vi "Set RAM and CPU Channel Properties.vi"(8 "error in (no error)":errorcluster, 10 "Logger Parameters":T1, 11 "Refnum in":refnum<k34>) -> (0 "error out":errorcluster, 3 "Refnum out":refnum<k34>)   [LabVIEW 2019, in "Telemetry Engine.lvlib"]
doc: "This VI sets the Physical Memory and CPU channel information along with their properties."
uses:
  Telemetry Engine.lvlib
  Types/Logger Data.ctl
  Types/Async Logger State Data.ctl
  Types/System Channels.ctl
  Types/Target Info.ctl
  Shared/Constants.vi
  Shared/Telemetry Shared.lvlib
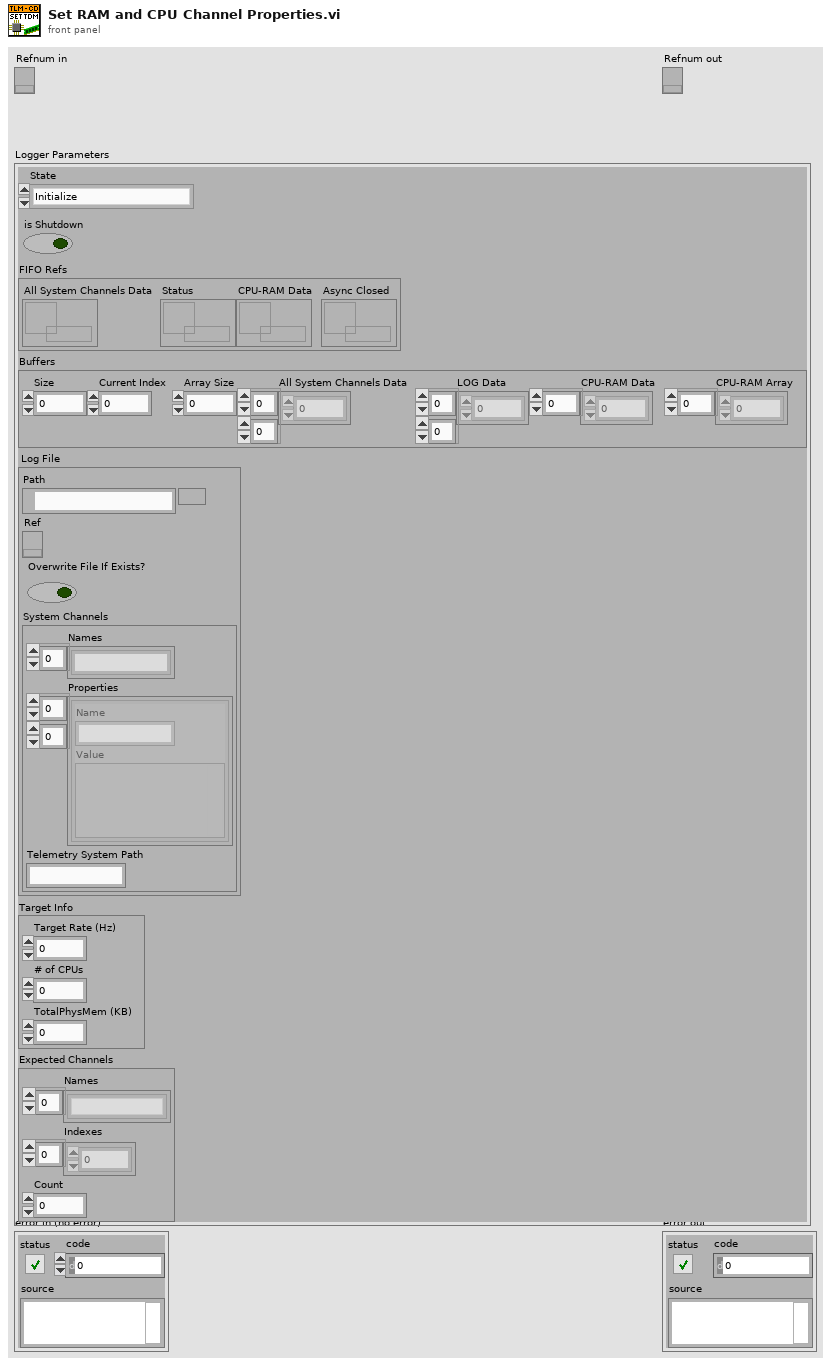
[diagram p1: front panel]
types:
  T1 = typedef "Telemetry Engine.lvlib/Logger Data.ctl" = cluster{"State":T2, "is Shutdown":bool, "FIFO Refs":cluster{"All System Channels Data":refnum<k33>, "Status":refnum<k33>, "CPU-RAM Data":refnum<k33>, "Async Closed":refnum<k33>}, "Buffers":cluster{"Size":i32, "Current Index":i32, "Array Size":i32, "All System Channels Data":dbl[][], "LOG Data":dbl[][], "CPU-RAM Data":dbl[], "CPU-RAM Array":dbl[]}, "Log File":cluster{"Path":path, "Ref":refnum<k34>, "Overwrite File If Exists?":bool, "System Channels":T3}, "Target Info":T4, "Expected Channels":cluster{"Names":string[], "Indexes":i32[], "Count":i32}}
  T2 = typedef "Telemetry Engine.lvlib/Async Logger State Data.ctl" = enum16{"Initialize", "Read System Channels FIFO", "Filter System Channels", "Read CPU-RAM FIFO", "Log Data", "Shutdown"}
  T3 = typedef "Telemetry Engine.lvlib/System Channels.ctl" = cluster{"Names":string[], "Properties":cluster{"Name":string, "Value":variant}[][], "Telemetry System Path":string}
  T4 = typedef "Telemetry Engine.lvlib/Target Info.ctl" = cluster{"Target Rate (Hz)":dbl, "# of CPUs":u32, "TotalPhysMem (KB)":dbl}
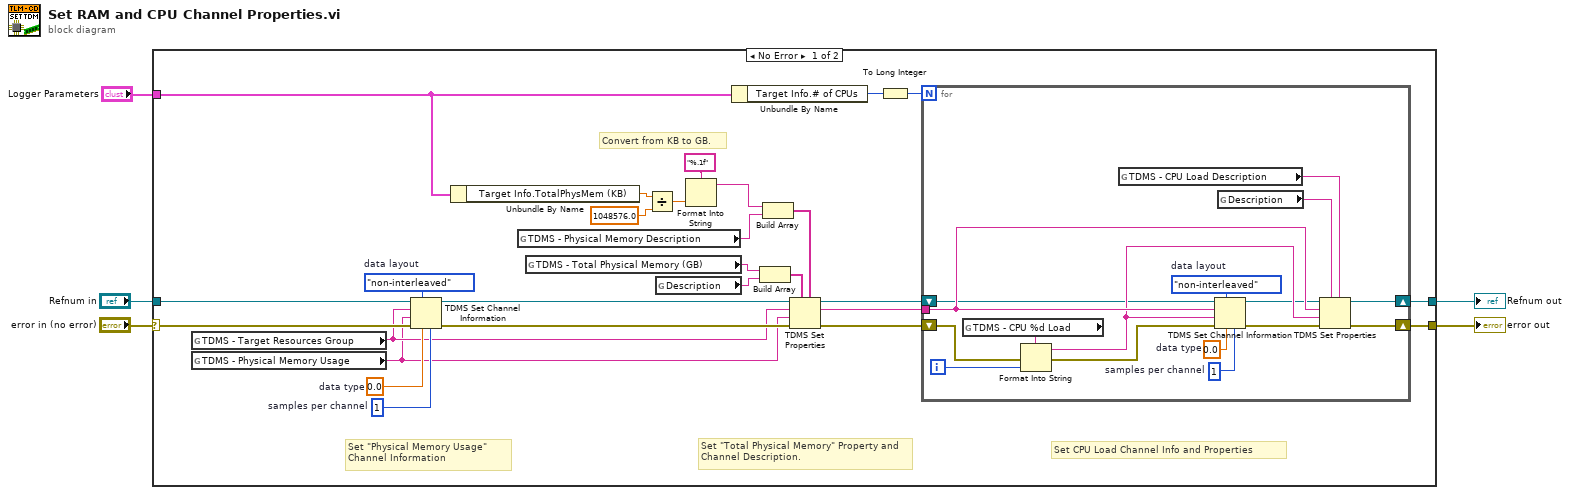
[diagram p0: block diagram]
diagram:
  n1 = case shown="No Error" "error in (no error)" {
    selector: "error in (no error)" -> [w28 w50]
    tunnel: "Logger Parameters" -> [w21 _]
    tunnel: "Refnum in" -> [w26 w49]
    tunnel: [w18 w49] -> w4
    tunnel: [w22 w50] -> w3
    frame No Error {
      w23 = u32 1  # samples per channel
      w24 = 0.0  # data type
      w25 = enum16{"non-interleaved", "interleaved"}."non-interleaved"  # data layout
      # "Set CPU Load Channel Info and Properties"
      # "Set \"Physical Memory Usage\" Channel Information"
      # "Set \"Total Physical Memory\" Property and Channel Description."
      # "Convert from KB to GB."
      n2 = global read "Constants.vi" "TDMS - Target Resources Group"() -> (w7:string)
      n3 = global read "Constants.vi" "TDMS - Physical Memory Usage"() -> (w6:string)
      n4 = TDMS Set Channel Information(4:w23, 6:w24, 7:w25, 8:w28, 9:w6, 10:w7, 11:w26) -> (0:w29:errorcluster, 3:w27:refnum<k34>)
      n5 = Unbundle By Name(w21) -> ("Target Info.TotalPhysMem (KB)"=w31:dbl)
      n6 = global read "Constants.vi" "TDMS - Physical Memory Description"() -> (w11:string)
      n7 = global read "Constants.vi" "TDMS - Total Physical Memory (GB)"() -> (w14:string)
      n8 = Divide(x=w31, y=1048576.0) -> (x/y=w17:dbl)
      n9 = global read "Constants.vi" "Description"() -> (w12:string)
      n10 = Format Into String(format string="%.1f", w17) -> (resulting string=w13:string)  [unwired: 2 in, 1 out]
      n11 = Unbundle By Name(w21) -> ("Target Info.# of CPUs"=w20:u32)
      n12 = Build Array(w14, w12) -> (w15:string[])
      n13 = Build Array(w13, w11) -> (w10:string[])
      n14 = TDMS Set Properties(5:w10, 7:w15, 8:w29, 9:w6, 10:w7, 11:w27) -> (0:w32:errorcluster, 2:w9:string, 3:w8:refnum<k34>)  [unwired: 1 out]
      n15 = To Long Integer(number=w20) -> (32bit integer=w19:i32)
      n16 = for {
        N: w19 -> [_]
        shift-right: [w47] -> w22
        shift-left: w32 -> [w43]
        tunnel: w9 -> [w40]
        shift-right: [w36] -> w18
        shift-left: w8 -> [w38]
        i -> [w41]
        w44 = enum16{"non-interleaved", "interleaved"}."non-interleaved"  # data layout
        w45 = 0.0  # data type
        w46 = u32 1  # samples per channel
        n17 = global read "Constants.vi" "TDMS - CPU %d Load"() -> (w33:string)
        n18 = Format Into String(format string=w33, error in=w43, w41) -> (resulting string=w39:string, error out=w42:errorcluster)  [unwired: 1 in]
        n19 = global read "Constants.vi" "TDMS - CPU Load Description"() -> (w34:string)
        n20 = TDMS Set Channel Information(4:w46, 6:w45, 7:w44, 8:w42, 9:w39, 10:w40, 11:w38) -> (0:w48:errorcluster, 3:w37:refnum<k34>)
        n21 = global read "Constants.vi" "Description"() -> (w35:string)
        n22 = TDMS Set Properties(5:w34, 7:w35, 8:w48, 9:w39, 10:w40, 11:w37) -> (0:w47:errorcluster, 3:w36:refnum<k34>)  [unwired: 2 out]
      }
    }
    frame Error {
    }
  }
  "Refnum out" <- w4
  "error out" <- w3
